vi "GyroCalculation.vi"(1 "NavX Enable":bool) -> (0 "Yaw":dbl)   [LabVIEW 2018]
uses:
  <vilib>/Rock Robotics/Network Tables/NT Write Number.vi
  <vilib>/Rock Robotics/Network Tables/NT Write Boolean.vi
panel:
  out "YRPHfH":T1
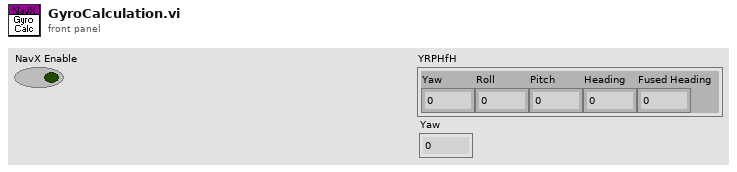
[diagram p1: front panel]
types:
  T1 = cluster{"Yaw":dbl, "Roll":dbl, "Pitch":dbl, "Heading":dbl, "Fused Heading":dbl}
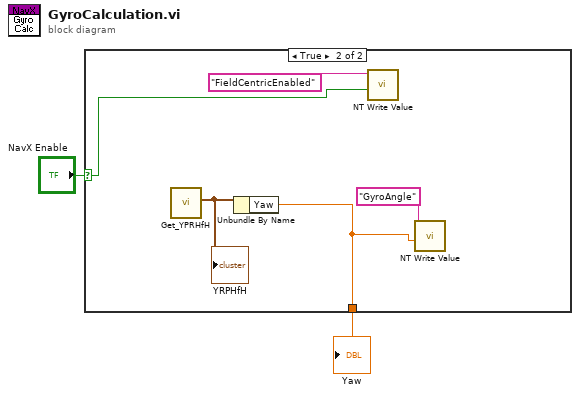
[diagram p0: block diagram]
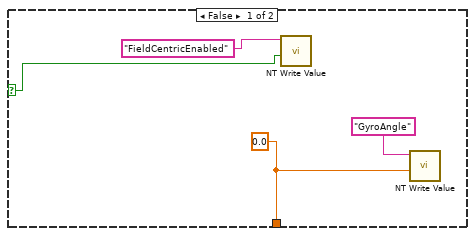
[diagram p2: hidden frame]
diagram:
  n1 = case shown="True" "NavX Enable" {
    selector: "NavX Enable" -> [w6 w7]
    tunnel: [w3 w10] -> w1
    frame False {
      w3 = 0.0
      n2 = call-poly <vilib>:"NT Write Value.vi"("Boolean"=w6, "Name"="FieldCentricEnabled") -> ()  [unwired: 9 in, 1 out]
      n3 = call-poly <vilib>:"NT Write Value.vi"("Numeric"=w3, "Name"="GyroAngle") -> ()  [unwired: 9 in, 1 out]
    }
    frame True {
      n4 = call <vilib>:"Get_YPRHfH.vi"() -> ("YRPHfH"=w11:T1)  [unwired: 11 in]
      "YRPHfH" <- w11
      n5 = Unbundle By Name(w11) -> ("Yaw"=w10:dbl)
      n6 = call-poly <vilib>:"NT Write Value.vi"("Boolean"=w7, "Name"="FieldCentricEnabled") -> ()  [unwired: 9 in, 1 out]
      n7 = call-poly <vilib>:"NT Write Value.vi"("Numeric"=w10, "Name"="GyroAngle") -> ()  [unwired: 9 in, 1 out]
    }
  }
  "Yaw" <- w1
